vi "Stop Core.vi"(10 "final error code":i32, 11 "Alpha in":refnum<class "Alpha.lvclass">) -> (3 "Alpha out":refnum<class "Alpha.lvclass">)   [LabVIEW 2017, in "Alpha Actor.lvlib" / "Alpha.lvclass"]
uses:
  Alpha.lvclass
  <vilib>/ActorFramework/Time-Delayed Send Message/Time-Delay Override Options.ctl
  Alpha.lvclass/Alpha.ctl
  <vilib>/ActorFramework/Actor/Actor.lvclass
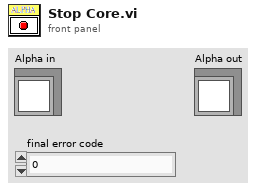
[diagram p1: front panel]
types:
  T1 = typedef "Time-Delay Override Options.ctl" = enum16{"Send next copy now", "Skip next scheduled copy", "Send next copy now and stop all further copies", "Stop all further copies"}
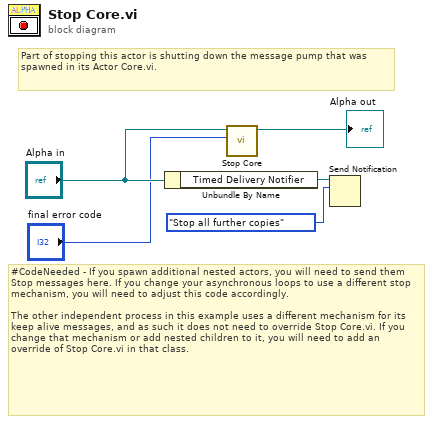
[diagram p0: block diagram]
diagram:
  # "#CodeNeeded - If you spawn additional nested actors, you will need to send them Stop messages here. If you change your asynchronous loops to use a different stop mechanism, you will need to adjust this code accordingly.\n\nThe other independent process in this example uses a different mechanism for its keep alive messages, and as such it does not need to override Stop Core.vi. If you change that mechanism or add nested children to it, you will need to add an override of Stop Core.vi in that class."
  # "Part of stopping this actor is shutting down the message pump that was spawned in its Actor Core.vi."
  n1 = Unbundle By Name("Alpha in") -> ("Timed Delivery Notifier"=w3:refnum<notifier>)
  n2 = call-parent "Stop Core.vi"("final error code"="final error code", "Actor in"="Alpha in") -> ("Actor out"=→"Alpha out":refnum<class "Alpha.lvclass">)  [unwired: 9 in]
  n3 = Send Notification(notification=Time-Delay_Override_Options."Stop all further copies", notifier=w3) -> ()  [unwired: 1 in, 2 out]
